vi "ConvTableTlog.vi"(2 "Mesure":dbl=2252.74, 3 "Courbe conversion":u16(ring) items=["Aucune conversion", "DT-670 Lakeshore", "DT-470 Lakeshore", "Ro600 Lakeshore", "CX-1010 Lakeshore", "CX-1010-Cu", "Ruo600A", "RO600A 2894", "Allen Bradley Res", "CX1050-Cu x38077", "CX1050-Cu x44121"]) -> (0 "Température":dbl=0.30718483818544784 format="%.4f", 1 "Courbe conv":refnum<vi>)   [LabVIEW 2010]
panel:
  in  "Tableau Calibrations":cluster{"Sensor":dbl, "Kelvin":dbl}[][](array[cluster])=array11x578[6358 elements]
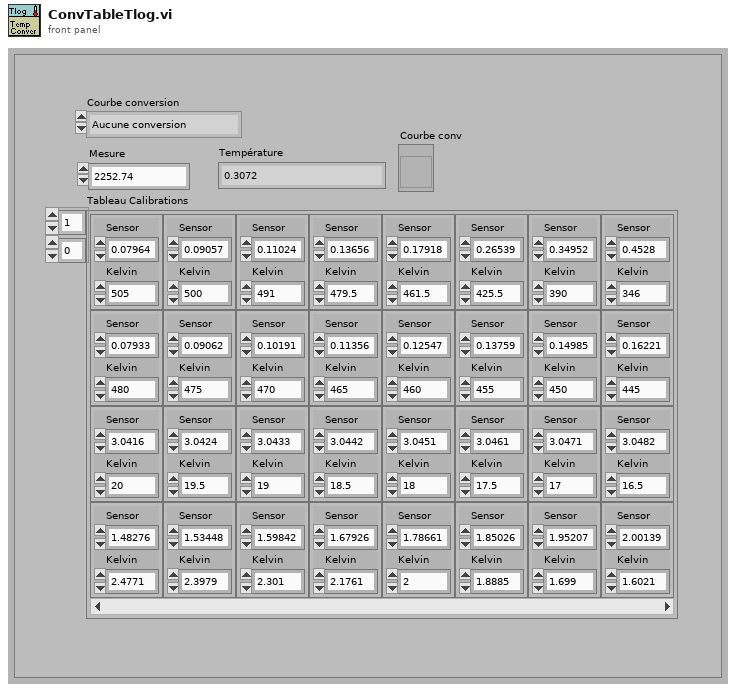
[diagram p1: front panel]
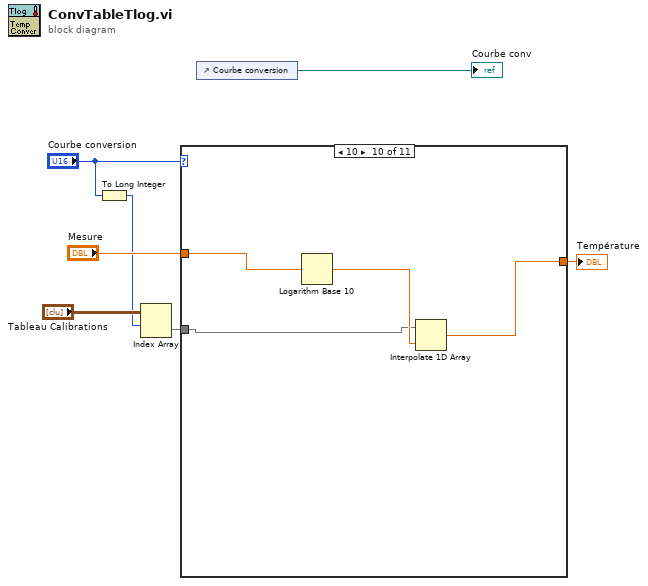
[diagram p0: block diagram]
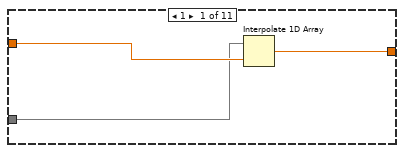
[diagram p2: hidden frame]
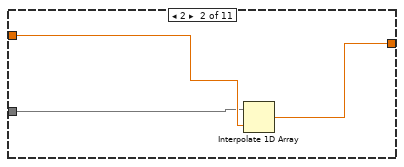
[diagram p3: hidden frame]
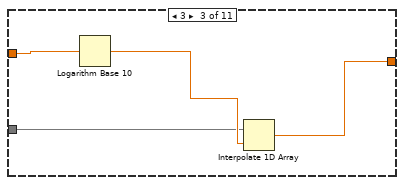
[diagram p4: hidden frame]
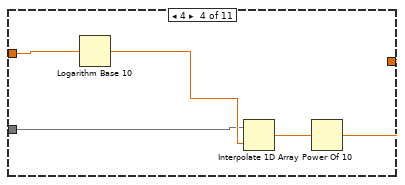
[diagram p5: hidden frame]
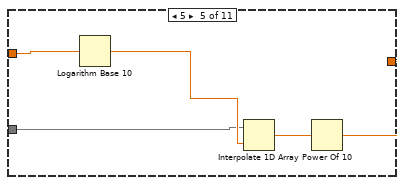
[diagram p6: hidden frame]
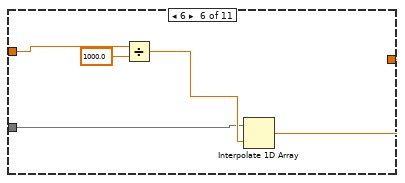
[diagram p7: hidden frame]
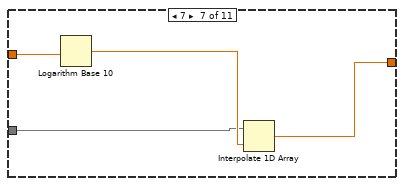
[diagram p8: hidden frame]
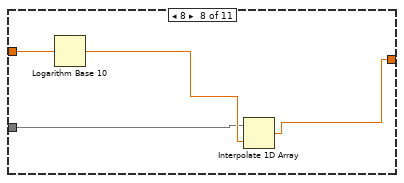
[diagram p9: hidden frame]
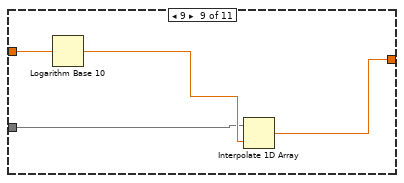
[diagram p10: hidden frame]
diagram:
  n1 = To Long Integer(number="Courbe conversion") -> (32bit integer=w1:i32)
  n2 = Index Array(array="Tableau Calibrations", index (row)=w1) -> (element=w2:cluster{"Sensor":dbl, "Kelvin":dbl}[])  [unwired: 1 in]
  n3 = case shown="10" "Courbe conversion" {
    tunnel: "Mesure" -> [w10 w13 w16 w22 w27 w31 w35 w40 w44 w48 w49]
    tunnel: [w9 w12 w17 w19 w24 w32 w36 w39 w43 w46 w49] -> w5
    tunnel: w2 -> [w8 w11 w14 w18 w23 w28 w33 w37 w41 w45 _]
    frame 1 {
      n4 = Interpolate 1D Array(1:w10, 2:w8) -> (0:w9:dbl)
    }
    frame 2 {
      n5 = Interpolate 1D Array(1:w13, 2:w11) -> (0:w12:dbl)
    }
    frame 3 {
      n6 = Logarithm Base 10(1:w16) -> (0:w15:dbl)
      n7 = Interpolate 1D Array(1:w15, 2:w14) -> (0:w17:dbl)
    }
    frame 4 {
      n8 = Logarithm Base 10(1:w22) -> (0:w21:dbl)
      n9 = Interpolate 1D Array(1:w21, 2:w18) -> (0:w20:dbl)
      n10 = Power Of 10(x=w20) -> (10^x=w19:dbl)
    }
    frame 5 {
      n11 = Logarithm Base 10(1:w27) -> (0:w26:dbl)
      n12 = Interpolate 1D Array(1:w26, 2:w23) -> (0:w25:dbl)
      n13 = Power Of 10(x=w25) -> (10^x=w24:dbl)
    }
    frame 6 {
      n14 = Divide(x=w31, y=1000.0) -> (x/y=w30:dbl)
      n15 = Interpolate 1D Array(1:w30, 2:w28) -> (0:w32:dbl)
    }
    frame 7 {
      n16 = Logarithm Base 10(1:w35) -> (0:w34:dbl)
      n17 = Interpolate 1D Array(1:w34, 2:w33) -> (0:w36:dbl)
    }
    frame 8 {
      n18 = Logarithm Base 10(1:w40) -> (0:w38:dbl)
      n19 = Interpolate 1D Array(1:w38, 2:w37) -> (0:w39:dbl)
    }
    frame 9 {
      n20 = Logarithm Base 10(1:w44) -> (0:w42:dbl)
      n21 = Interpolate 1D Array(1:w42, 2:w41) -> (0:w43:dbl)
    }
    frame 10 {
      n22 = Logarithm Base 10(1:w48) -> (0:w47:dbl)
      n23 = Interpolate 1D Array(1:w47, 2:w45) -> (0:w46:dbl)
    }
    frame 0, Default {
    }
  }
  "Température" <- w5
  n24 = control-ref of="Courbe conversion"() -> (→"Courbe conv":refnum<vi>)
